vi "Finished Collection Write File.vi"(6 "Cluster in":T1, 9 "Corrected Array in":dbl[][](array[numeric]), 10 "Feet of\nStainless to be\nUsed (Count) in":i32, 11 "Output KPRO":path=path "c:/junk.dat") -> (1 "Corrected Array out":dbl[][](array[numeric]), 2 "Depth to \nbe Used \n(Feet)":sgl, 3 "Feet of\nStainless to be\nUsed (Count) out":i32)   [LabVIEW 2016]
uses:
  controls/Kpro hydraulic measurement cluster.ctl
  <vilib>/Utility/file.llb/Write Delimited Spreadsheet (DBL).vi
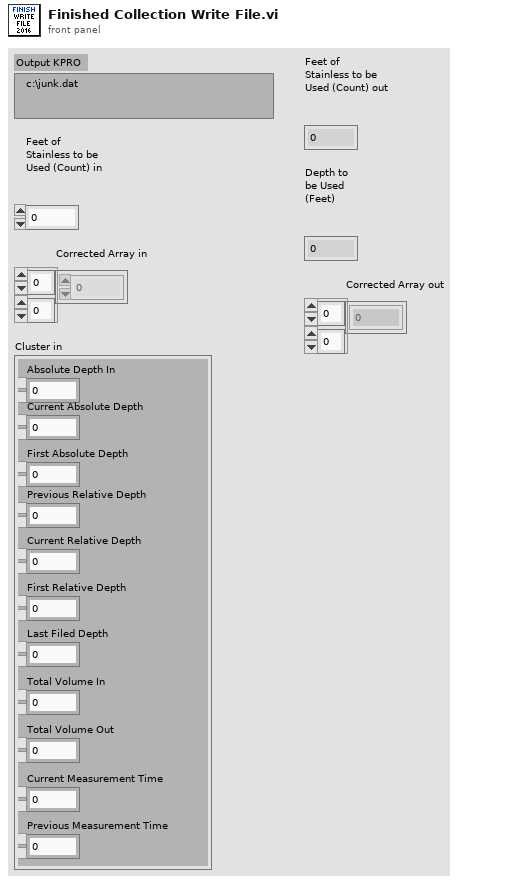
[diagram p1: front panel]
types:
  T1 = typedef "Kpro hydraulic measurement cluster.ctl" = cluster{"Absolute Depth In":dbl, "Current Absolute Depth":dbl, "First Absolute Depth":dbl, "Previous Relative Depth":dbl, "Current Relative Depth":dbl, "First Relative Depth":dbl, "Last Filed Depth":dbl, "Total Volume In":dbl, "Total Volume Out":dbl, "Current Measurement Time":dbl, "Previous Measurement Time":dbl}
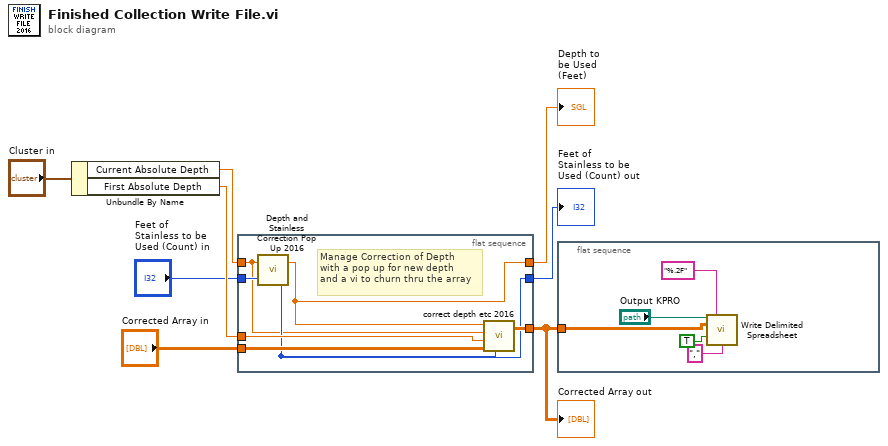
[diagram p0: block diagram]
diagram:
  n1 = Unbundle By Name("Cluster in") -> ("Current Absolute Depth"=w7:dbl, "First Absolute Depth"=w8:dbl)
  n2 = flat-sequence {
    tunnel: "Corrected Array in" -> [w15]
    tunnel: [w14] -> w2
    tunnel: w8 -> [w13]
    tunnel: [w12] -> w3
    tunnel: "Feet of\nStainless to be\nUsed (Count) in" -> [w11]
    tunnel: [w10] -> w5
    tunnel: w7 -> [w9]
    frame #0 {
      # "Manage Correction of Depth\nwith a pop up for new depth\nand a vi to churn thru the array"
      n3 = call "Depth and Stainless Correction Pop Up 2016.vi"("New Number\n of Stainless\n(Count)"=w11, "Input \nCorrected \nDepth (Feet)"=w9) -> ("Feet of\nStainless to be\nUsed (Count)"=w10:i32, "Depth to \nbe Used \n(Feet)"=w14:sgl)
      n4 = call "correct depth etc 2016.vi"("Correct Depth"=w14, "Incorrect Depth"=w9, "First Absolute Depth"=w13, "Uncorrected Array"=w15, "New Stainless Feet"=w10) -> ("Corrected Array"=w12:dbl[][])  [unwired: 1 in]
    }
  }
  n5 = flat-sequence {
    tunnel: w3 -> [w19]
    frame #0 {
      n6 = call-poly <vilib>:"Write Delimited Spreadsheet.vi"("file path (dialog if empty)"="Output KPRO", "format (%.3f)"="%.2F", "2D data"=w19, "append to file? (new file:F)"=TRUE, "delimiter (\\t)"="," ("delimiter (\\t)")) -> ()  [unwired: 9 in, 2 out]
    }
  }
  "Feet of\nStainless to be\nUsed (Count) out" <- w5
  "Corrected Array out" <- w3
  "Depth to \nbe Used \n(Feet)" <- w2
